vi "430_TCP_Query (multiple commands).vi"(7 "Number of\nquerys":i32, 8 "error in (no error)":errorcluster, 9 "Timeout":i32=1000, 10 "Command":string, 11 "connection ID":refnum<k5>) -> (0 "error out":errorcluster, 1 "Bytes Read":i32, 2 "Response":string, 3 "connection ID out":refnum<k5>, 4 "Bytes Written":i32)   [LabVIEW 2011]
panel:
  in  "error out 3":errorcluster
  out "error out 2":errorcluster
  out "data out":string
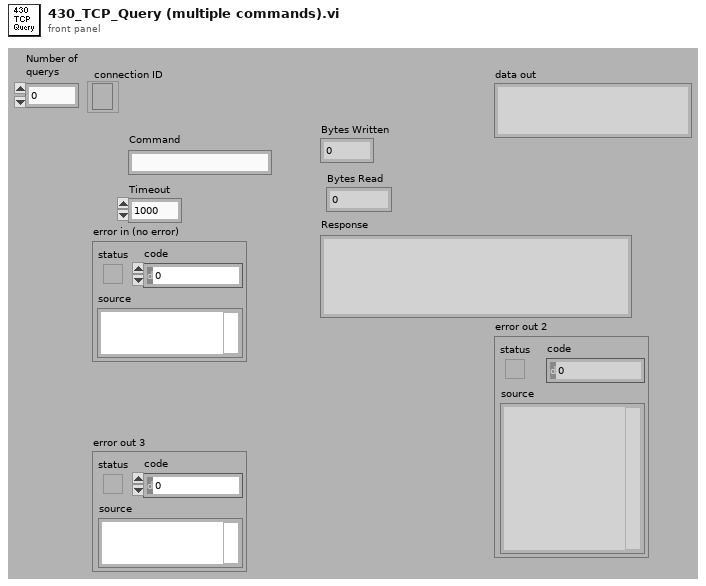
[diagram p1: front panel]
types:
  T1 = enum16{"Standard", "Buffered", "CRLF", "Immediate"}
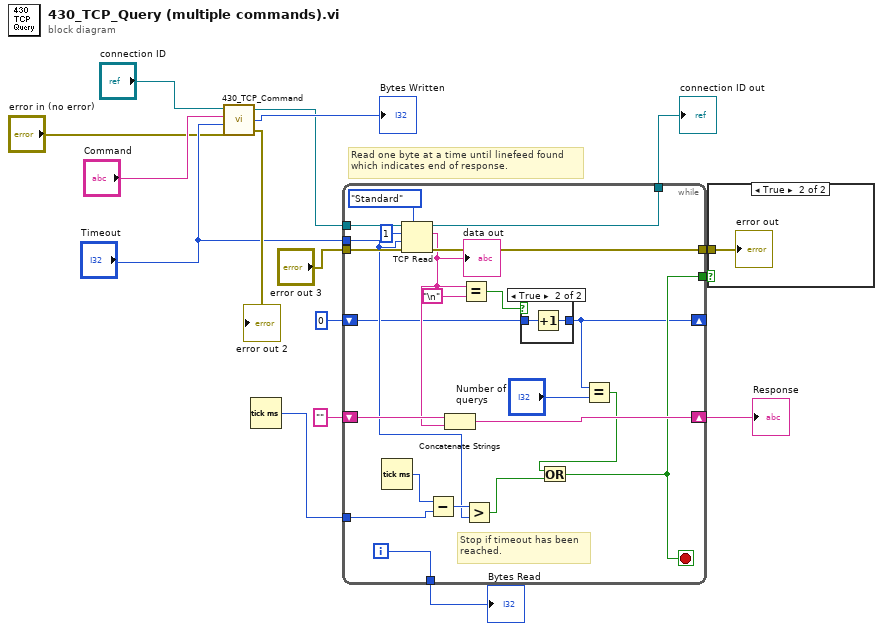
[diagram p0: block diagram]
diagram:
  # "Read one byte at a time until linefeed found\nwhich indicates end of response."
  n1 = call "430_TCP_Command.vi"("error in (no error)"="error in (no error)", "Timeout"="Timeout", "Command"="Command", "connection ID"="connection ID") -> ("error out"=→"error out 2":errorcluster, "bytes written"=→"Bytes Written":i32, "connection ID out"=w14:refnum<k5>)
  n2 = Tick Count (ms)() -> (millisecond timer value=w7:u32)
  n3 = while {
    tunnel: w14 -> [w38]
    tunnel: [w37] -> w13
    tunnel: "error out 3" -> [w36]
    tunnel: [w35] -> w11
    tunnel: [w34] -> w10
    shift-right: [w28] -> w8
    shift-left: "" -> [w30]
    tunnel: "Timeout" -> [w23]
    tunnel: w7 -> [w26]
    tunnel: [w22] -> w6
    shift-right: [w18] -> _
    shift-left: 0 -> [w19]
    i -> [w34]
    stop <- w22 stop-if-true
    # "Stop if timeout has been\nreached."
    n4 = Tick Count (ms)() -> (millisecond timer value=w27:u32)
    n5 = TCP Read(connection ID=w38, bytes to read=1, error in (no error)=w36, 7:T1."Standard" ("mode (standard)"), 9:w23) -> (connection ID out=w37:refnum<k5>, data out=w29:string, error out=w35:errorcluster)
    "data out" <- w29
    n6 = Subtract(x=w27, y=w26) -> (x-y=w25:u32)
    n7 = Concatenate Strings(w30, w29) -> (w28:string)
    n8 = Equal?(x=w29, y="\n") -> (x = y?=w21:bool)
    n9 = Greater?(x=w25, y=w23) -> (0:w24:bool)
    n10 = case shown="True" w21 {
      tunnel: w19 -> [w39 w40]
      tunnel: [w39 w41] -> w18
      frame False {
      }
      frame True {
        n11 = Increment(x=w40) -> (x+1=w41:i32)
      }
    }
    n12 = Equal?(x=w18, y="Number of\nquerys") -> (x = y?=w20:bool)
    n13 = Or(x=w20, y=w24) -> (x .or. y?=w22:bool)
  }
  "Bytes Read" <- w10
  "Response" <- w8
  "connection ID out" <- w13
  n14 = case shown="True" w6 {
    tunnel: w11 -> [_ w42]
    frame False {
    }
    frame True {
      "error out" <- w42
    }
  }
